vi "niScope Read Cluster.vi"(7 "timeout":dbl=5.0 format="%.2f", 8 "error in":errorcluster, 9 "numSamples":i32=-1, 10 "channels":string="0", 11 "instrument handle":refnum<k15>) -> (0 "error out":errorcluster, 1 "waveform":T2 {"wfm" format="%.2f"; "xIncrement" format="%.2f"; "relativeInitialX" format="%.2f"}, 2 "wfm info":T1 {"reserved2" format="%.2f"; "reserved1" format="%.2f"; "offset" format="%^.3e"; "gain" format="%^.3e"; "xIncrement" format="%^.3e"; "relativeInitialX" format="%^.3e"; "absoluteInitialX" format="%^.3e"}, 3 "instrument handle out":refnum<k15>)   [LabVIEW 2013]
doc: "Initiates an acquisition, waits for it to complete, and retrieves the data for a single channel and record."
uses:
  niScope_32.dll
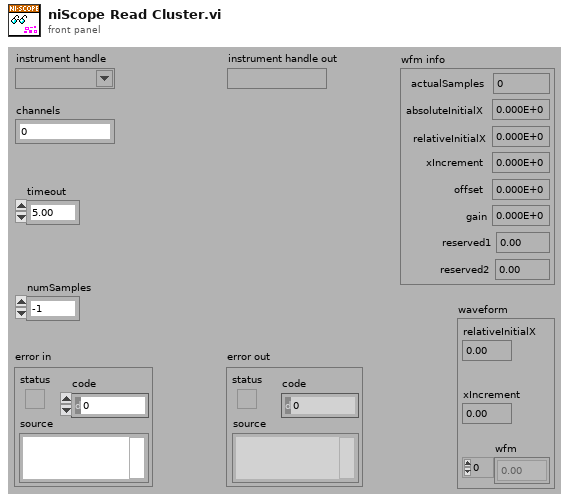
[diagram p1: front panel]
types:
  T1 = cluster{"actualSamples":i32, "absoluteInitialX":dbl, "relativeInitialX":dbl, "xIncrement":dbl, "offset":dbl, "gain":dbl, "reserved1":dbl, "reserved2":dbl}
  T2 = cluster{"relativeInitialX":dbl, "xIncrement":dbl, "wfm":dbl[]}
  T3 = cluster{"Element Data":dbl, "Element Data":dbl, dbl[]}
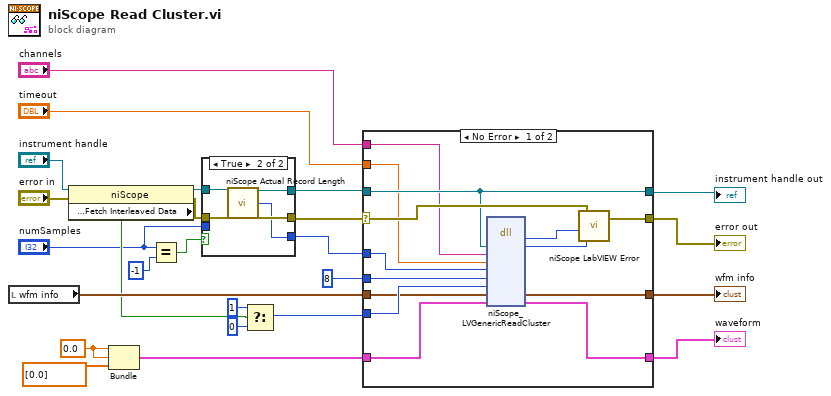
[diagram p0: block diagram]
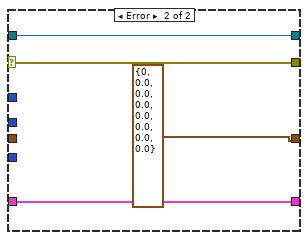
[diagram p2: hidden frame]
diagram:
  w18 = 0.0 ("Element Data")
  n1 = local read "wfm info"() -> (w22:T1)
  n2 = property class="niScope"(reference="instrument handle", error in="error in") -> (reference out=w12:refnum<k15>, error out=w13:errorcluster, "Device Specific:IF Digitizer (5620 and 5621):Advanced:Fetch Interleaved Data"=w14:bool)
  n3 = Bundle("Element Data"=w18, "Element Data"=w18, dbl[] [0.0]) -> (w20:T3)  [unwired: 1 in]
  n4 = Equal?(x="numSamples", y=-1) -> (x = y?=w4:bool)
  n5 = case shown="True" w4 {
    tunnel: [w27 w33] -> w16
    tunnel: [w28 w32] -> w6
    tunnel: "numSamples" -> [w26 _]
    tunnel: [w26 w29] -> w21
    tunnel: w12 -> [w28 w31]
    tunnel: w13 -> [w27 w30]
    frame False {
    }
    frame True {
      n6 = call <instrlib>:"niScope Actual Record Length.vi"("instrument handle"=w31, "error in"=w30) -> ("instrument handle out"=w32:refnum<k15>, "actual record length"=w29:i32, "error out"=w33:errorcluster)  [unwired: 11 in]
    }
  }
  n7 = Select(t=1, s=w14, f=0) -> (s? t:f=w15:i32)
  n8 = case shown="No Error" w16 {
    selector: w16 -> [w44 w50]
    tunnel: [w45 w50] -> w1
    tunnel: w6 -> [w43 w51]
    tunnel: [w43 w51] -> w2
    tunnel: w21 -> [w34 _]
    tunnel: [w40 T1 {"actualSamples"=0, "absoluteInitialX"=0.0, "relativeInitialX"=0.0, "xIncrement"=0.0, "offset"=0.0, "gain"=0.0, "reserved1"=0.0, "reserved2"=0.0}] -> w7
    tunnel: w15 -> [w39 _]
    tunnel: [w41 w49] -> w17
    tunnel: w20 -> [w42 w49]
    tunnel: w22 -> [w38 _]
    tunnel: 8 ("dataType") -> [w37 _]
    tunnel: "timeout" -> [w36 _]
    tunnel: "channels" -> [w35 _]
    frame No Error {
      n9 = dll-call lib="niScope_*.*" fn="niScope_LVGenericReadCluster"("instrument handle"=w43, "channel"=w35, "timeout"=w36, "numSamples"=w34, "dataType"=w37, "interleaved"=w39, "wfm_info"=w38, "in_cluster"=w42) -> ("status"=w47:i32, "instrument handle"=w46:u32, "wfm_info"=w40:T1, "in_cluster"=w41:T3)  [unwired: 8 in, 2 out]
      n10 = call <instrlib>:"niScope LabVIEW Error.vi"("instrument handle"=w46, "niScope error code (0)"=w47, "error in (no error)"=w44) -> ("error out"=w45:errorcluster)  [unwired: 2 in]
    }
    frame Error {
    }
  }
  "waveform" <- w17
  "wfm info" <- w7
  "error out" <- w1
  "instrument handle out" <- w2
